vi "FGV GD Errors sammeln.vi"(6 "Aktion":T4, 7 "Sprachliste":string[][](array[string]), 8 "error in (no error)":errorcluster caption="Fehler (Eingang, kein Fehler)", 10 "Kalibrier Info-Cluster in":T1, 11 "GD Info-Cluster in":T2) -> (0 "error out":errorcluster caption="Fehler (Ausgang)", 2 "Kalibrier Info-Cluster out":T1[](array[typedef]), 3 "GD Info-Cluster out":T2[](array[typedef]))   [LabVIEW 2020, in "Linearisierung v2.lvlib" / "SpanEinstellungen.lvlib"]
uses:
  SpanEinstellungen.lvlib
  Aktion FGV GD Errors sammeln.ctl
  GD Info Cluster.ctl
  LIN ErrorCluster.ctl
  Kalibrier Info Cluster.ctl
  Linearisierung v2.lvlib
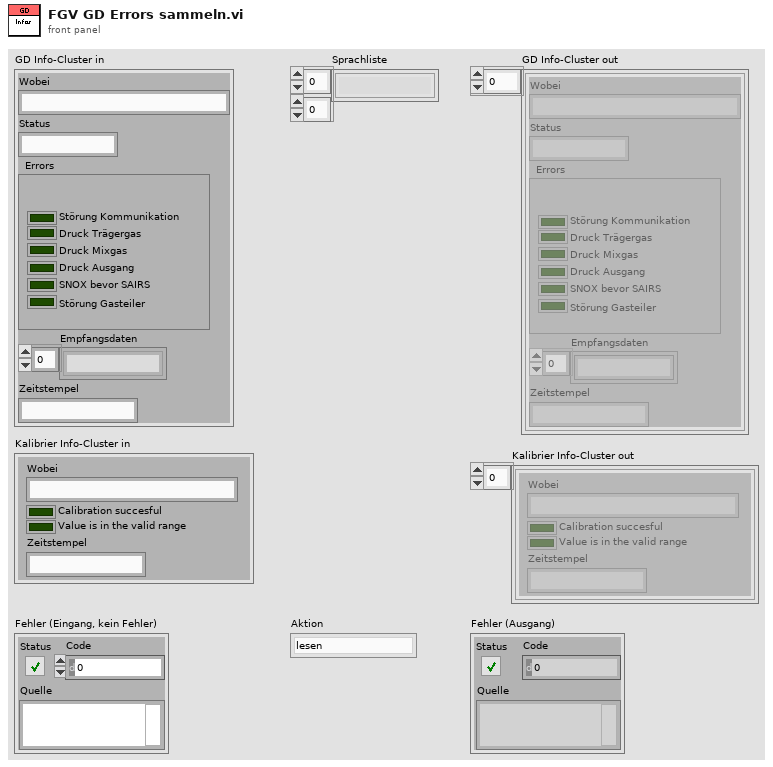
[diagram p1: front panel]
types:
  T1 = typedef "Linearisierung v2.lvlib/SpanEinstellungen.lvlib/Kalibrier Info Cluster.ctl" = cluster{"Wobei":string, "Calibration succesful":bool, "Value is in the valid range":bool, "Zeitstempel":string}
  T2 = typedef "Linearisierung v2.lvlib/SpanEinstellungen.lvlib/GD Info Cluster.ctl" = cluster{"Wobei":string, "Status":string, "Errors":T3, "Empfangsdaten":string[], "Zeitstempel":string}
  T3 = typedef "Linearisierung v2.lvlib/LIN ErrorCluster.ctl" = cluster{"Störung Kommunikation":bool, "Pressure carrier gas":bool, "Pressure diluted gas":bool, "Outlet Pressure":bool, "SNOX before SAIR":bool, "Störung Gasteiler":bool}
  T4 = typedef "Linearisierung v2.lvlib/SpanEinstellungen.lvlib/Aktion FGV GD Errors sammeln.ctl" = enum16{"lesen", "init", "GD Infos sammeln", "Kalibrierinfos sammeln", "Test Data", "GD Infos selektiv sammeln"}
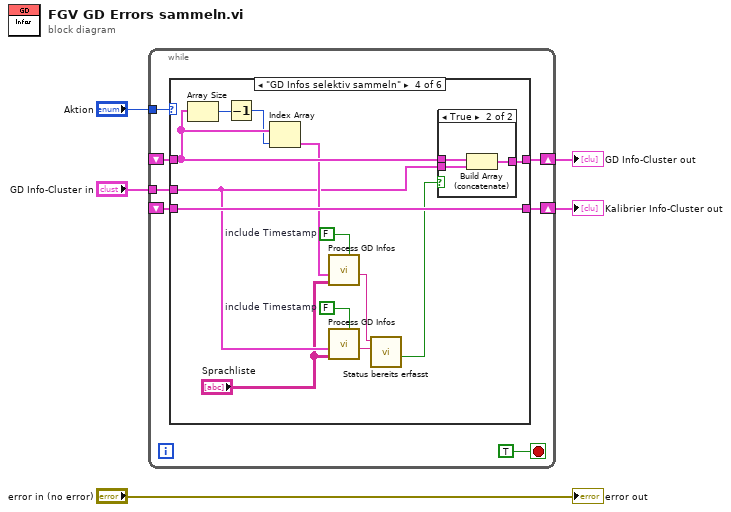
[diagram p0: block diagram]
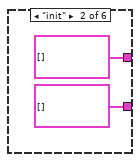
[diagram p3: hidden frame]
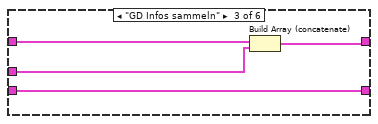
[diagram p4: hidden frame]
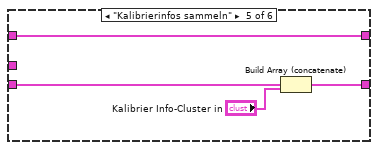
[diagram p6: hidden frame]
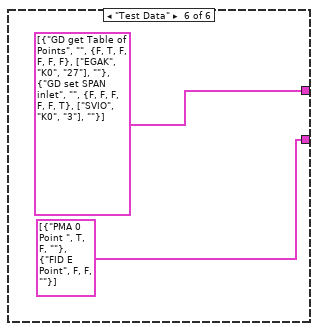
[diagram p7: hidden frame]
diagram:
  n1 = while {
    tunnel: "Aktion" -> [w12]
    shift-right: [w10] -> w4
    shift-left: _ -> [w9]
    shift-right: [w8] -> w2
    shift-left: _ -> [w7]
    tunnel: "GD Info-Cluster in" -> [w6]
    stop <- TRUE stop-if-true
    n2 = case shown="\"GD Infos selektiv sammeln\"" w12 {
      tunnel: [w14 T2[] [] ("GD Info-Cluster in") w19 w33 w41 T2[] [{"Wobei"="GD get Table of Points", "Status"="", "Errors"={"Störung Kommunikation"=FALSE, "Pressure carrier gas"=TRUE, "Pressure diluted gas"=FALSE, "Outlet Pressure"=FALSE, "SNOX before SAIR"=FALSE, "Störung Gasteiler"=FALSE}, "Empfangsdaten"=["EGAK", "K0", "27"], "Zeitstempel"=""}, {"Wobei"="GD set SPAN inlet", "Status"="", "Errors"={"Störung Kommunikation"=FALSE, "Pressure carrier gas"=FALSE, "Pressure diluted gas"=FALSE, "Outlet Pressure"=FALSE, "SNOX before SAIR"=FALSE, "Störung Gasteiler"=TRUE}, "Empfangsdaten"=["SVIO", "K0", "3"], "Zeitstempel"=""}] ("GD Info-Cluster in")] -> w10
      tunnel: w9 -> [w14 _ w20 w29 w41 _]
      tunnel: [w13 T1[] [] ("Array") w18 w32 w39 T1[] [{"Wobei"="PMA 0 Point ", "Calibration succesful"=TRUE, "Value is in the valid range"=FALSE, "Zeitstempel"=""}, {"Wobei"="FID E Point", "Calibration succesful"=FALSE, "Value is in the valid range"=FALSE, "Zeitstempel"=""}] ("Array")] -> w8
      tunnel: w7 -> [w13 _ w18 w32 w38 _]
      tunnel: w6 -> [_ _ w17 w24 _ _]
      frame "lesen", Default {
      }
      frame "init" {
      }
      frame "GD Infos sammeln" {
        n3 = Build Array (concatenate)(w20, w17) -> (w19:T2[])
      }
      frame "GD Infos selektiv sammeln" {
        w28 = FALSE  # include Timestamp
        w31 = FALSE  # include Timestamp
        n4 = Array Size(array=w29) -> (size(s)=w23:i32)
        n5 = Decrement(x=w23) -> (x-1=w22:i32)
        n6 = Index Array(array=w29, index=w22) -> (element=w27:T2)
        n7 = call "Process GD Infos.vi"("include Timestamp"=w28, "Sprachliste"="Sprachliste", "GD Info-Cluster in"=w27) -> ("GD Infos"=w26:string)  [unwired: 6 in, 2 out]
        n8 = call "Process GD Infos.vi"("include Timestamp"=w31, "Sprachliste"="Sprachliste", "GD Info-Cluster in"=w24) -> ("GD Infos"=w30:string)  [unwired: 6 in, 2 out]
        n9 = call "Status bereits erfasst.vi"("Status new in"=w30, "Status old in"=w26) -> ("unique"=w25:bool)  [unwired: 6 in, 3 out]
        n10 = case shown="True" w25 {
          tunnel: [w34 w37] -> w33
          tunnel: w29 -> [w34 w36]
          tunnel: w24 -> [_ w35]
          frame False {
          }
          frame True {
            n11 = Build Array (concatenate)(w36, w35) -> (w37:T2[])
          }
        }
      }
      frame "Kalibrierinfos sammeln" {
        n12 = Build Array (concatenate)(w38, "Kalibrier Info-Cluster in") -> (w39:T1[])
      }
      frame "Test Data" {
      }
    }
  }
  "GD Info-Cluster out" <- w4
  "Kalibrier Info-Cluster out" <- w2
  "error out" <- "error in (no error)"
